vi "Write lvlibretls server listener.vi"(10 "lvlibretls server listener":refnum<class "lvlibretls server listener.lvclass">, 11 "TLS HTTP handler dataset in":refnum<class "TLS HTTP handler dataset.lvclass">) -> (3 "TLS HTTP handler dataset out":refnum<class "TLS HTTP handler dataset.lvclass">)   [LabVIEW 2016]
uses:
  TLS HTTP handler dataset.lvclass
  C:/Users/IEUser/Desktop/http/HTTP handler dataset/basic HTTP handler dataset.lvclass
  lvlibtls/server/lvlibretls server listener.lvclass
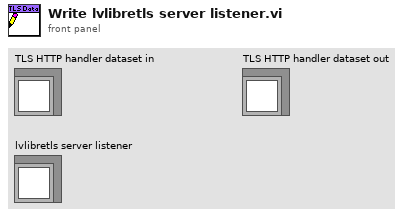
[diagram p1: front panel]
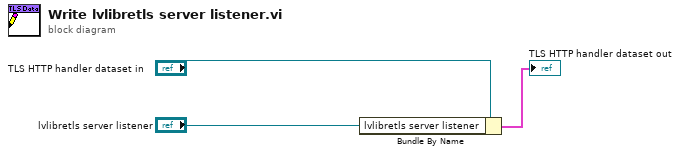
[diagram p0: block diagram]
diagram:
  n1 = Bundle By Name(cluster="TLS HTTP handler dataset in", "lvlibretls server listener"="lvlibretls server listener") -> (→"TLS HTTP handler dataset out":cluster{})
